vi "Analysis.Indicate Filterd Result Summary Item.vi"(10 "Filters":T2 {"Date2" items=["2019-01-01"]; "Date1" items=["2019-01-01"]}, 11 "ResultSum":T1) -> (3 "In Filter":bool)   [LabVIEW 2024]
uses:
  Analysis.Result Summary Filters.ctl
  Analysis.Result Summary.ctl
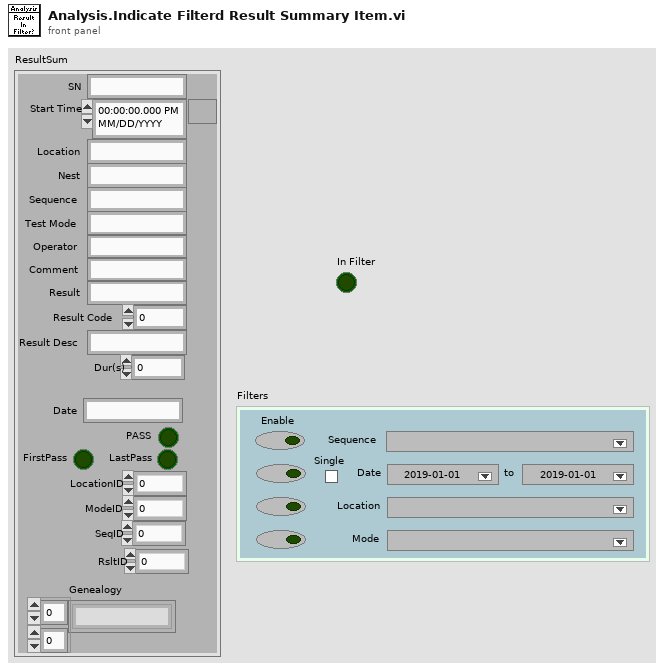
[diagram p1: front panel]
types:
  T1 = typedef "Analysis.Result Summary.ctl" = cluster{"SN":string, "Start Time":timestamp, "Location":string, "Nest":string, "Sequence":string, "Operator":string, "Test Mode":string, "Comment":string, "Result":string, "Result Code":i32, "Result Desc":string, "Date":string, "Dur(s)":dbl, "PASS":bool, "FirstPass":bool, "LastPass":bool, "LocationID":i32, "ModeID":i32, "SeqID":i32, "RsltID":i32, "Genealogy":string[][]}
  T2 = typedef "Analysis.Result Summary Filters.ctl" = cluster{"Filter En Seq":bool, "Sequence":u16, "Filter En Date":bool, "Date1":u16, "Location":u16, "Filter En Loc":bool, "Mode":u16, "Filter En Mode":bool, "Seq List":string[], "Date List":string[], "Loc List":string[], "Mode List":string[], "Date2":u16, "Date Range":bool}
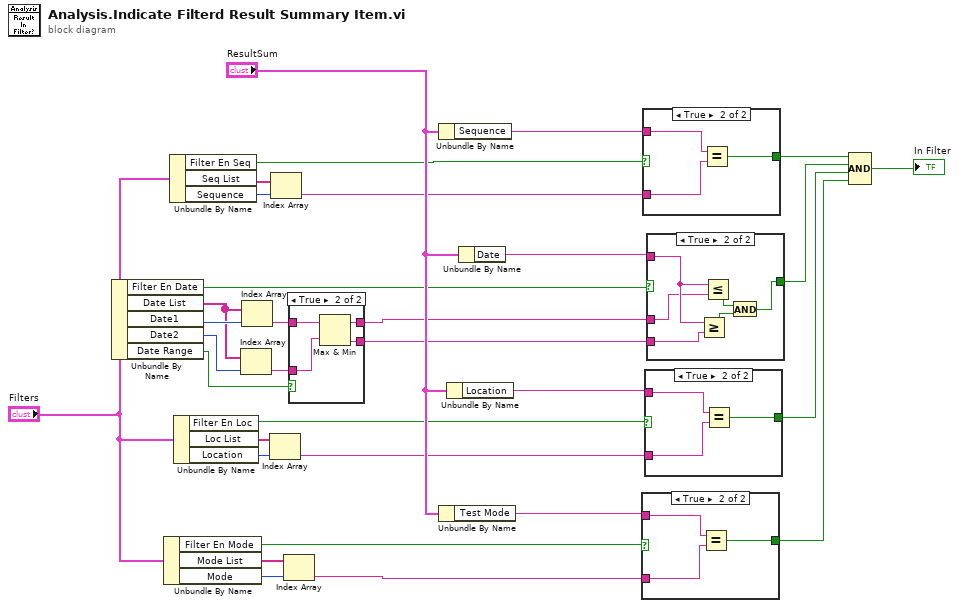
[diagram p0: block diagram]
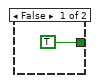
[diagram p2: hidden frame]
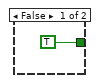
[diagram p3: hidden frame]
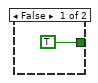
[diagram p4: hidden frame]
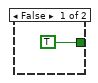
[diagram p5: hidden frame]
diagram:
  n1 = Unbundle By Name("Filters") -> ("Filter En Date"=w30:bool, "Date List"=w16:string[], "Date1"=w31:u16, "Date2"=w15:u16, "Date Range"=w10:bool)
  n2 = Unbundle By Name("Filters") -> ("Filter En Mode"=w19:bool, "Mode List"=w24:string[], "Mode"=w23:u16)
  n3 = Unbundle By Name("Filters") -> ("Filter En Seq"=w26:bool, "Seq List"=w28:string[], "Sequence"=w29:u16)
  n4 = Unbundle By Name("Filters") -> ("Filter En Loc"=w18:bool, "Loc List"=w25:string[], "Location"=w22:u16)
  n5 = Index Array(array=w16, index=w15) -> (element=w13:string)
  n6 = Index Array(array=w16, index=w31) -> (element=w14:string)
  n7 = Index Array(array=w25, index=w22) -> (element=w21:string)
  n8 = Index Array(array=w28, index=w29) -> (element=w27:string)
  n9 = Index Array(array=w24, index=w23) -> (element=w20:string)
  n10 = case shown="True" w10 {
    tunnel: w14 -> [w33 w37]
    tunnel: w13 -> [_ w36]
    tunnel: [w33 w35] -> w12
    tunnel: [w33 w34] -> w11
    frame False {
    }
    frame True {
      n11 = Max & Min(x=w37, y=w36) -> (max(x,y)=w35:string, min(x,y)=w34:string)
    }
  }
  n12 = Unbundle By Name("ResultSum") -> ("Sequence"=w9:string)
  n13 = Unbundle By Name("ResultSum") -> ("Test Mode"=w5:string)
  n14 = Unbundle By Name("ResultSum") -> ("Location"=w6:string)
  n15 = Unbundle By Name("ResultSum") -> ("Date"=w7:string)
  n16 = case shown="True" w19 {
    tunnel: w5 -> [_ w41]
    tunnel: w20 -> [_ w40]
    tunnel: [TRUE w39] -> w2
    frame False {
    }
    frame True {
      n17 = Equal?(x=w41, y=w40) -> (x = y?=w39:bool)
    }
  }
  n18 = case shown="True" w26 {
    tunnel: w9 -> [_ w45]
    tunnel: w27 -> [_ w44]
    tunnel: [TRUE w43] -> w8
    frame False {
    }
    frame True {
      n19 = Equal?(x=w45, y=w44) -> (x = y?=w43:bool)
    }
  }
  n20 = case shown="True" w18 {
    tunnel: w6 -> [_ w49]
    tunnel: w21 -> [_ w48]
    tunnel: [TRUE w47] -> w3
    frame False {
    }
    frame True {
      n21 = Equal?(x=w49, y=w48) -> (x = y?=w47:bool)
    }
  }
  n22 = case shown="True" w30 {
    tunnel: w7 -> [_ w52]
    tunnel: w12 -> [_ w51]
    tunnel: [TRUE w54] -> w4
    tunnel: w11 -> [_ w56]
    frame False {
    }
    frame True {
      n23 = Greater Or Equal?(x=w52, y=w56) -> (x >= y?=w55:bool)
      n24 = Less Or Equal?(x=w52, y=w51) -> (x <= y?=w53:bool)
      n25 = And(x=w53, y=w55) -> (x .and. y?=w54:bool)
    }
  }
  n26 = Compound Arithmetic op=AND(w8, w4, w3, w2) -> (→"In Filter":bool)
